vi "Radians to Degrees.vi"   [LabVIEW 2017, in "NI_AngleConversion.lvlib"]
doc: "Converts data from radians to degrees."
uses:
  <vilib>/Analysis/NI_AngleConversion.lvlib
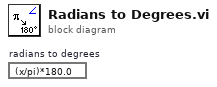
[diagram p0: block diagram]
diagram:
  n1 = expression code="(x/pi)*180.0" "radians to degrees"() -> ()  [unwired: 1 in, 1 out]
